vi "Resolve Glyph.vi"(7 "Size":dbl=16.0, 8 "error in (no error)":errorcluster, 10 "Glyph Name":string, 11 "Glyph Source in":refnum<class "Glyph Source.lvclass">) -> (0 "error out":errorcluster, 1 "charcode":u32, 2 "Font":refnum<class "Font Settings.lvclass">, 3 "Glyph Source out":refnum<class "Glyph Source.lvclass">)   [LabVIEW 2023, in "Font Glyph Drawer Interface.lvlib" / "Glyph Source.lvclass"]
uses:
  Glyph Source.lvclass
  Font Settings/Font Settings.lvclass
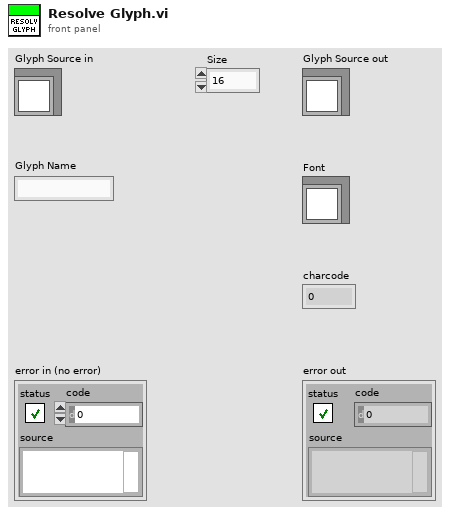
[diagram p1: front panel]
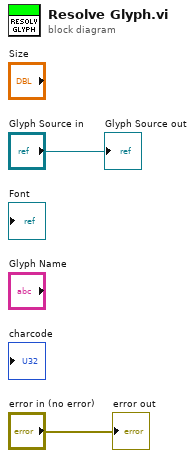
[diagram p0: block diagram]
diagram:
  "error out" <- "error in (no error)"
  "Glyph Source out" <- "Glyph Source in"
